vi "putForceActuatorData.vi"(8 "error in (no error)":errorcluster, 10 "TelemetryForceActuatorData":T1, 11 "M1M3SAL in":refnum<class "M1M3SAL.lvclass">) -> (0 "error out":errorcluster, 3 "M1M3SAL out":refnum<class "M1M3SAL.lvclass">)   [LabVIEW 2016, in "M1M3SupportCommunicator.lvlib" / "M1M3SAL.lvclass"]
uses:
  M1M3SAL.lvclass
  DataTypes/Topics/TelemetryForceActuatorData.ctl
  DataTypes/Topics/Parts/Timestamp.ctl
  DataTypes/MessageHeader.ctl
  DataTypes/MessageTypes.ctl
  DataTypes/MessageTopics.ctl
  Common_RT_Utilities/U8ArrayBuilderAutoIndexing/U8ArrayBuilderAutoIndexing.lvclass
  M1M3SupportCommunicator.lvlib
  DataTypes/Topics/M1M3SupportTopics.lvlib
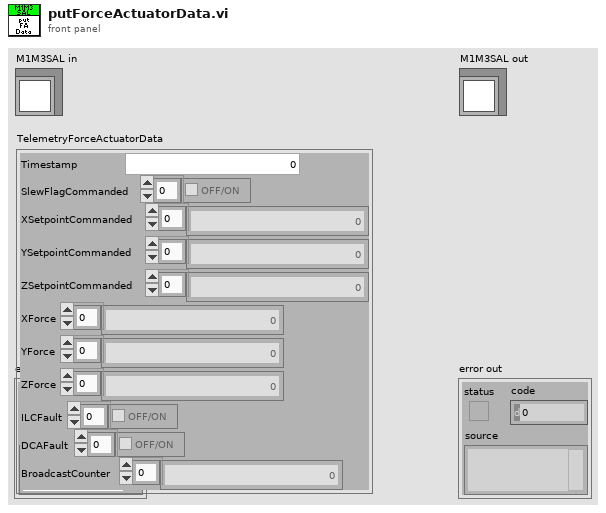
[diagram p1: front panel]
types:
  T1 = typedef "M1M3SupportTopics.lvlib/TelemetryForceActuatorData.ctl" = cluster{"Timestamp":T2, "SlewFlagCommanded":bool[], "XSetpointCommanded":dbl[], "YSetpointCommanded":dbl[], "ZSetpointCommanded":dbl[], "XForce":sgl[], "YForce":sgl[], "ZForce":sgl[], "ILCFault":bool[], "DCAFault":bool[], "BroadcastCounter":u8[]}
  T2 = typedef "M1M3SupportTopics.lvlib/Timestamp.ctl" = dbl
  T3 = typedef "M1M3SupportCommunicator.lvlib/MessageHeader.ctl" = cluster{"Type":T4, "Topic":T5, "Size":i32}
  T4 = typedef "M1M3SupportCommunicator.lvlib/MessageTypes.ctl" = enum8{"None", "PutSample", "GetNextSample", "LogEvent", "GetEvent", "IssueCommand", "CommandId", "WaitForCompletion", "AcceptCommand", "AckCommand"}
  T5 = typedef "M1M3SupportCommunicator.lvlib/MessageTopics.ctl" = enum8{"None", "ForceActuatorData", "MirrorForceData", "HardpointData", "AirData", "DynamicData", "FPGAData", "IMSData", "ForceActuatorStatus", "ElevationData", "HardpointStatus", "HardpointActuatorChase", "AirStatus", "ForceActuatorSafetyChecks", "ForceActuatorTest", "ActuatorBroadcastCounter", "StatusChecks", "CellChecks", "HardpointActuatorBreakaway", "RaiseMirrorComplete", "ILCCommunication", "ElevationAngleChecks", "DetailedState", "ServoLoops", "ForceActuatorInfo", "LowerMirrorComplete", "HardpointActuatorInfo", "SettingsApplied", "ErrorCode", "StartupChecks", "SummaryState", "SettingVersions", "ActuatorTestStatus", "AppliedSettingsMatchStart", "Enable", "EnterMaintenance", "Standby", "AbortLowerM1M3", "ApplyAberrationByForces", "ApplyAOSCorrectionByBendingModes", "ClearAOSCorrection", "Start", "RaiseM1M3", "TestForceActuator", "LowerM1M3", "ApplyAOSCorrectionByForces", "Disable", "ApplyAberationByBendingMode", "TestHardpoint", "ManipulateM1M3", "ClearAberration", "Exit", "TestAir", "AbortRaiseM1M3", "MoveHardpointActuators", "ExitMaintenance", "Shutdown"}
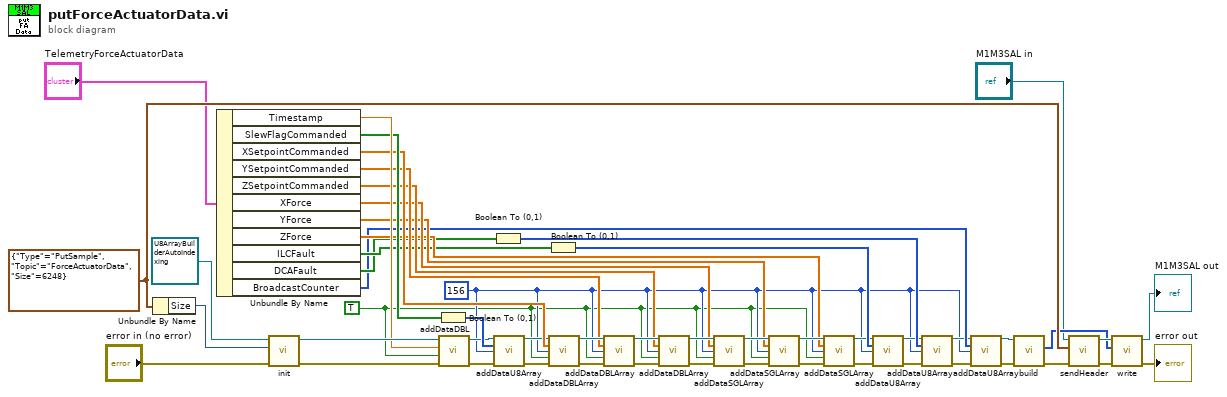
[diagram p0: block diagram]
diagram:
  w1 = TRUE ("OverrideSwapBytes")
  w7 = 156 ("Length")
  w51 = T3 {"Type"=enum."PutSample", "Topic"=enum."ForceActuatorData", "Size"=6248} ("MessageHeader")
  n1 = Unbundle By Name(w51) -> ("Size"=w50:i32)
  n2 = Unbundle By Name("TelemetryForceActuatorData") -> ("Timestamp"=w39:T2, "SlewFlagCommanded"=w37:bool[], "XSetpointCommanded"=w33:dbl[], "YSetpointCommanded"=w28:dbl[], "ZSetpointCommanded"=w26:dbl[], "XForce"=w23:sgl[], "YForce"=w20:sgl[], "ZForce"=w17:sgl[], "ILCFault"=w15:bool[], "DCAFault"=w12:bool[], "BroadcastCounter"=w9:u8[])
  n3 = call "init.vi"("error in (no error)"="error in (no error)", "Size"=w50, "U8ArrayBuilderAutoIndexing in"=refnum<class "U8ArrayBuilderAutoIndexing.lvclass"> refnum ("RTUtilities.lvlib:U8ArrayBuilderAutoIndexing.lvclass")) -> ("error out"=w38:errorcluster, "U8ArrayBuilderAutoIndexing out"=w40:refnum<class "U8ArrayBuilderAutoIndexing.lvclass">)  [unwired: 7 in]
  n4 = Boolean To (0,1)(Boolean=w37) -> (0, 1=w36:i16[])
  n5 = call "addDataDBL.vi"("error in (no error)"=w38, "OverrideSwapBytes"=w1, "Data"=w39, "U8ArrayBuilderAutoIndexing in"=w40) -> ("error out"=w34:errorcluster, "U8ArrayBuilderAutoIndexing out"=w35:refnum<class "U8ArrayBuilderAutoIndexing.lvclass">)  [unwired: 6 in]
  n6 = Boolean To (0,1)(Boolean=w12) -> (0, 1=w13:i16[])
  n7 = call "addDataU8Array.vi"("U8ArrayBuilderAutoIndexing in"=w35, "Data"=w36, "Length"=w7, "error in (no error)"=w34) -> ("U8ArrayBuilderAutoIndexing out"=w32:refnum<class "U8ArrayBuilderAutoIndexing.lvclass">, "error out"=w31:errorcluster)  [unwired: 10 in]
  n8 = Boolean To (0,1)(Boolean=w15) -> (0, 1=w14:i16[])
  n9 = call "addDataDBLArray.vi"("U8ArrayBuilderAutoIndexing in"=w32, "Data"=w33, "Length"=w7, "OverrideSwapBytes"=w1, "error in (no error)"=w31) -> ("U8ArrayBuilderAutoIndexing out"=w30:refnum<class "U8ArrayBuilderAutoIndexing.lvclass">, "error out"=w29:errorcluster)  [unwired: 9 in]
  n10 = call "addDataDBLArray.vi"("U8ArrayBuilderAutoIndexing in"=w30, "Data"=w28, "Length"=w7, "OverrideSwapBytes"=w1, "error in (no error)"=w29) -> ("U8ArrayBuilderAutoIndexing out"=w27:refnum<class "U8ArrayBuilderAutoIndexing.lvclass">, "error out"=w25:errorcluster)  [unwired: 9 in]
  n11 = call "addDataDBLArray.vi"("U8ArrayBuilderAutoIndexing in"=w27, "Data"=w26, "Length"=w7, "OverrideSwapBytes"=w1, "error in (no error)"=w25) -> ("U8ArrayBuilderAutoIndexing out"=w24:refnum<class "U8ArrayBuilderAutoIndexing.lvclass">, "error out"=w22:errorcluster)  [unwired: 9 in]
  n12 = call "addDataSGLArray.vi"("U8ArrayBuilderAutoIndexing in"=w24, "Data"=w23, "Length"=w7, "OverrideSwapBytes"=w1, "error in (no error)"=w22) -> ("U8ArrayBuilderAutoIndexing out"=w21:refnum<class "U8ArrayBuilderAutoIndexing.lvclass">, "error out"=w19:errorcluster)  [unwired: 9 in]
  n13 = call "addDataSGLArray.vi"("U8ArrayBuilderAutoIndexing in"=w21, "Data"=w20, "Length"=w7, "OverrideSwapBytes"=w1, "error in (no error)"=w19) -> ("U8ArrayBuilderAutoIndexing out"=w18:refnum<class "U8ArrayBuilderAutoIndexing.lvclass">, "error out"=w16:errorcluster)  [unwired: 9 in]
  n14 = call "addDataSGLArray.vi"("U8ArrayBuilderAutoIndexing in"=w18, "Data"=w17, "Length"=w7, "OverrideSwapBytes"=w1, "error in (no error)"=w16) -> ("U8ArrayBuilderAutoIndexing out"=w11:refnum<class "U8ArrayBuilderAutoIndexing.lvclass">, "error out"=w6:errorcluster)  [unwired: 9 in]
  n15 = call "addDataU8Array.vi"("U8ArrayBuilderAutoIndexing in"=w11, "Data"=w14, "Length"=w7, "error in (no error)"=w6) -> ("U8ArrayBuilderAutoIndexing out"=w10:refnum<class "U8ArrayBuilderAutoIndexing.lvclass">, "error out"=w5:errorcluster)  [unwired: 10 in]
  n16 = call "addDataU8Array.vi"("U8ArrayBuilderAutoIndexing in"=w10, "Data"=w13, "Length"=w7, "error in (no error)"=w5) -> ("U8ArrayBuilderAutoIndexing out"=w8:refnum<class "U8ArrayBuilderAutoIndexing.lvclass">, "error out"=w4:errorcluster)  [unwired: 10 in]
  n17 = call "addDataU8Array.vi"("U8ArrayBuilderAutoIndexing in"=w8, "Data"=w9, "Length"=w7, "error in (no error)"=w4) -> ("U8ArrayBuilderAutoIndexing out"=w3:refnum<class "U8ArrayBuilderAutoIndexing.lvclass">, "error out"=w2:errorcluster)  [unwired: 10 in]
  n18 = call "build.vi"("error in (no error)"=w2, "U8ArrayBuilderAutoIndexing in"=w3) -> ("error out"=w47:errorcluster, "Array"=w48:u8[])  [unwired: 7 in, 1 out]
  n19 = call "sendHeader.vi"("error in (no error)"=w47, "MessageHeader"=w51, "M1M3SAL in"="M1M3SAL in") -> ("error out"=w46:errorcluster, "M1M3SAL out"=w49:refnum<class "M1M3SAL.lvclass">)  [unwired: 7 in]
  n20 = call "write.vi"("error in (no error)"=w46, "Data"=w48, "M1M3SAL in"=w49) -> ("error out"=→"error out":errorcluster, "M1M3SAL out"=→"M1M3SAL out":refnum<class "M1M3SAL.lvclass">)  [unwired: 7 in]
